vi "Write to Hardware.vi"(7 "Valid Triggers":bool, 8 "error in":errorcluster, 9 "Trigger Values":dbl[](array[numeric]), 10 "Values in":dbl[](array[numeric]), 11 "Tx Execution Unit Implementation in":refnum<class "Tx Generic Execution Unit.lvclass">) -> (0 "error out":errorcluster, 1 "Trigger Values out":dbl[](array[numeric]), 2 "Values out":dbl[](array[numeric]), 3 "Tx Execution Unit Implementation out":refnum<class "Tx Generic Execution Unit.lvclass">)   [LabVIEW 2020, in "AIM ARINC 664 Engine.lvlib" / "Implementation.lvlib" / "Tx Generic Execution Unit.lvclass"]
uses:
  Tx Generic Execution Unit.lvclass
  Tx Generic Execution Unit.lvclass/Tx Generic Execution Unit.ctl
  <instrlib>/AIM GmbH/_AIM 664/bsp/Fdx Stop (Tx).vi
  <instrlib>/AIM GmbH/_AIM 664/bsp/LIbraryAdmin/FdxGlobalDllPath.vi
  <instrlib>/AIM GmbH/_AIM 664/bsp/LIbraryAdmin/FdxGetErrorDescription.vi
  <vilib>/Utility/error.llb/Error Cluster From Error Code.vi
  <instrlib>/AIM GmbH/_AIM 664/AIM664LV.lvlib
  <vilib>/Utility/SystemLogging/NI_SystemLogging.lvlib
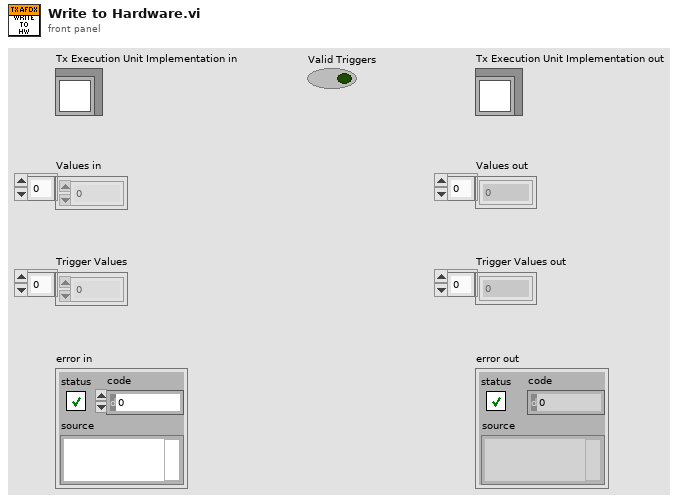
[diagram p1: front panel]
types:
  T1 = cluster{"StartMode":i32, "Count":u32, "Sign":i32, "Day":u32, "Hour":u32, "Min":u32, "Second":u32, "MilliSec":u32, "MicroSec":u32, "ExtendedStopMode":i32, "TransmitTime":u32}
  T2 = cluster{"Index":u32, "Offset":u32, "Lenght":u32, "SubQueueHandle":u32}
  T3 = typedef "Frame Payload Parameters.ctl" = cluster{"PayloadID":string, "FrameIndeces":u32[], "Parameters":cluster{"start index":i32, "size":i32, "encoding":T4, "signed":bool, "scale multiplier":dbl, "scale offset":dbl}[]}
  T4 = typedef "Encoding (Arinc664).ctl" = u16
  T5 = typedef "tx_generic_command.ctl" = enum16{"No Action", "Start", "Stop"}
  T6 = cluster{"start index":i32, "size":i32, "encoding":T4, "signed":bool, "scale multiplier":dbl, "scale offset":dbl}[]
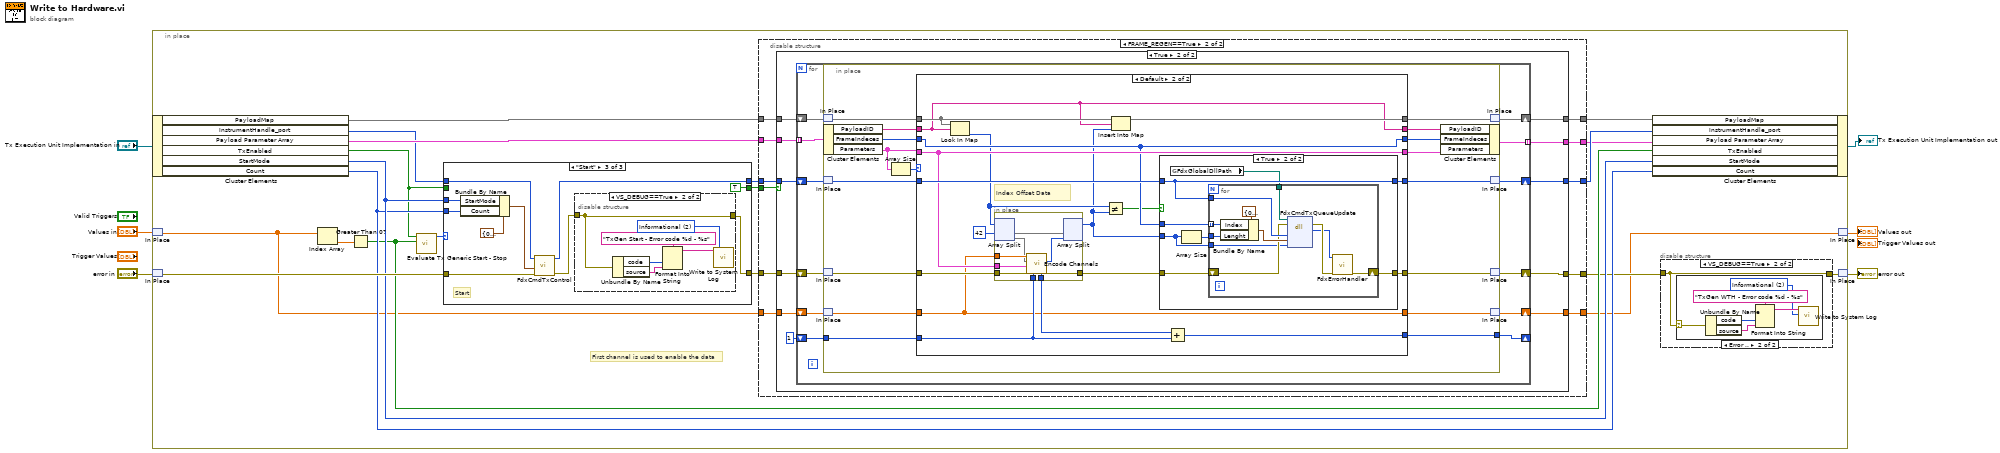
[diagram p0: block diagram]
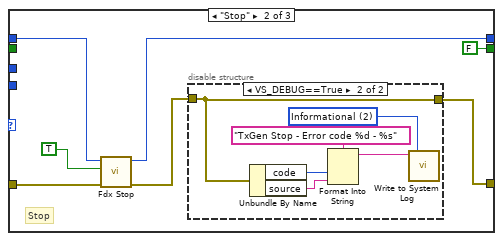
[diagram p5: hidden frame]
diagram:
  n1 = in-place {
    # "First channel is used to enable the data"
    n2 = in-place-cluster #1("Tx Execution Unit Implementation in") -> ("PayloadMap"=w8:map{string, u8[]}, "InstrumentHandle_port"=w22:u32, "Payload Parameter Array"=w26:T3[], "TxEnabled"=w11:bool, "StartMode"=w18:u32, "Count"=w17:u32)
    n3 = in-place-match #2("Values in") -> (w9:dbl[])
    n4 = in-place-match #3("error in") -> (w20:errorcluster)
    n5 = Index Array(array=w9) -> (element=w23:dbl)  [unwired: 1 in]
    n6 = Greater Than 0?(x=w23) -> (x > 0?=w15:bool)
    n7 = call "Evaluate Tx Generic Start - Stop.vi"("current"=w15, "last"=w11) -> ("tx generic command"=w16:T5)  [unwired: 9 in]
    n8 = case shown="\"Start\"" w16 {
      tunnel: w22 -> [w36 w41 w58]
      tunnel: w18 -> [_ _ w56]
      tunnel: w17 -> [_ _ w55]
      tunnel: w20 -> [w37 w43 w59]
      tunnel: [w37 w39 w53] -> w19
      tunnel: [w36 w42 w57] -> w21
      tunnel: w11 -> [w35 _ _]
      tunnel: [w35 FALSE ("TxEnabled") TRUE ("TxEnabled")] -> w10
      frame "No Action", Default {
      }
      frame "Stop" {
        # "Stop"
        n9 = call-poly <instrlib>:"Fdx Stop.vi"("error in"=w43, "Force Stop?"=TRUE, "InstrumentHandle_port in"=w41) -> ("error out"=w40:errorcluster, "InstrumentHandle_port out"=w42:u32)  [unwired: 7 in]
        n10 = disable-structure shown="VS_DEBUG==True" {
          disable-tunnel: w40 -> [w45 w46]
          disable-tunnel: [w45 w46] -> w39
          frame condition #0 {
          }
          frame condition #1 (active) {
            w49 = 2 items=["Error", "Warning", "Informational"] ("severity")
            n11 = Unbundle By Name(w46) -> ("code"=w48:i32, "source"=w47:string)
            n12 = Format Into String(format string="TxGen Stop - Error code %d - %s", w48, w47) -> (resulting string=w50:string)  [unwired: 2 in, 1 out]
            n13 = call <vilib>:"Write to System Log.vi"("severity"=w49, "message"=w50) -> ()  [unwired: 9 in, 1 out]
          }
        }
      }
      frame "Start" {
        # "Start"
        n14 = Bundle By Name(cluster=T1 {"StartMode"=0, "Count"=0, "Sign"=0, "Day"=0, "Hour"=0, "Min"=0, "Second"=0, "MilliSec"=0, "MicroSec"=0, "ExtendedStopMode"=0, "TransmitTime"=0} ("TxControl"), "StartMode"=w56, "Count"=w55) -> (w61:T1)
        n15 = call <instrlib>:"FdxCmdTxControl.vi"("error in"=w59, "TxControl"=w61, "InstrumentHandle_port in"=w58) -> ("error out"=w54:errorcluster, "InstrumentHandle_port out"=w57:u32)  [unwired: 7 in]
        n16 = disable-structure shown="VS_DEBUG==True" {
          disable-tunnel: w54 -> [w62 w63]
          disable-tunnel: [w62 w63] -> w53
          frame condition #0 {
          }
          frame condition #1 (active) {
            w66 = 2 items=["Error", "Warning", "Informational"] ("severity")
            n17 = Unbundle By Name(w63) -> ("code"=w65:i32, "source"=w64:string)
            n18 = Format Into String(format string="TxGen Start - Error code %d - %s", w65, w64) -> (resulting string=w67:string)  [unwired: 2 in, 1 out]
            n19 = call <vilib>:"Write to System Log.vi"("severity"=w66, "message"=w67) -> ()  [unwired: 9 in, 1 out]
          }
        }
      }
    }
    n20 = disable-structure shown="FRAME_REGEN==True" {
      disable-tunnel: w21 -> [w71 w81]
      disable-tunnel: w26 -> [w72 w79]
      disable-tunnel: w19 -> [w70 w83]
      disable-tunnel: [w70 w82] -> w14
      disable-tunnel: [w71 w80] -> w25
      disable-tunnel: [w72 w78] -> w24
      disable-tunnel: w9 -> [w69 w77]
      disable-tunnel: [w69 w76] -> w12
      disable-tunnel: w10 -> [_ w75]
      disable-tunnel: w8 -> [_ w74]
      disable-tunnel: [_ w73] -> w7
      frame condition #0 {
      }
      frame condition #1 (active) {
        n21 = case shown="True" w75 {
          tunnel: w83 -> [w86 w99]
          tunnel: [w86 w98] -> w82
          tunnel: w81 -> [w87 w97]
          tunnel: [w87 w96] -> w80
          tunnel: w79 -> [w88 w95]
          tunnel: [w88 w94] -> w78
          tunnel: w77 -> [w85 w89]
          tunnel: [w85 w93] -> w76
          tunnel: w74 -> [w84 w90]
          tunnel: [w84 w91] -> w73
          frame False {
          }
          frame True {
            n22 = for {
              shift-right: [w107] -> w98
              shift-left: w99 -> [w111]
              shift-right: [w104] -> w96
              shift-left: w97 -> [w110]
              tunnel: w95 -> [w109] mode=indexing
              tunnel: [w108] -> w94 mode=indexing
              shift-right: [w105] -> w93
              shift-left: w89 -> [w106]
              shift-right: [w103] -> _
              shift-left: 1 -> [w102]
              shift-right: [w101] -> w91
              shift-left: w90 -> [w100]
              n23 = in-place {
                in-place-border: [w125] -> w103
                in-place-border: w102 -> [w124]
                n24 = in-place-match #4(w100) -> (w121:map{string, u8[]})
                n25 = in-place-cluster #5(w109) -> ("PayloadID"=w119:string, "FrameIndeces"=w118:u32[], "Parameters"=w117:T6)
                n26 = in-place-match #6(w110) -> (w127:u32)
                n27 = in-place-match #7(w111) -> (w123:errorcluster)
                n28 = in-place-match #8(w106) -> (w126:dbl[])
                n29 = Array Size(array=w117) -> (size(s)=w122:i32)
                n30 = case shown="Default" w122 {
                  tunnel: [w136 w154] -> w128
                  tunnel: w127 -> [w134 w147]
                  tunnel: w126 -> [w129 w142]
                  tunnel: [w135 w152] -> w125
                  tunnel: w124 -> [w135 w151]
                  tunnel: w117 -> [w130 w144]
                  tunnel: w123 -> [w136 w150]
                  tunnel: w119 -> [w132 w143]
                  tunnel: w118 -> [w131 w140]
                  tunnel: w121 -> [w133 w146]
                  tunnel: [w134 w141] -> w120
                  tunnel: [w133 w145] -> w116
                  tunnel: [w131 w140] -> w115
                  tunnel: [w132 w143] -> w114
                  tunnel: [w130 w144] -> w113
                  tunnel: [w129 w142] -> w112
                  frame 0 {
                  }
                  frame Default {
                    # "Index Offset Data"
                    n31 = Look In Map(map=w146, key=w143) -> (value=w139:u8[])  [unwired: 1 in, 1 out]
                    n32 = in-place {
                      in-place-border: w142 -> [w183]
                      in-place-border: [w182] -> w153
                      in-place-border: w151 -> [w181]
                      in-place-border: w144 -> [w180]
                      in-place-border: w150 -> [w179]
                      in-place-border: [w178] -> w149
                      n33 = in-place-split #9(w139, 42) -> (w177:u8[], w176:u8[])
                      n34 = call "Encode Channels.vi"("Offset"=w181, "error in"=w179, "Parameters"=w180, "Data in"=w176, "Values in"=w183) -> ("error out"=w178:errorcluster, "Data out"=w175:u8[], "Number of Parameters"=w182:i32)  [unwired: 4 in]
                      n35 = in-place-split #9(w177, w175) -> (w138:u8[])  [unwired: 1 out]
                    }
                    n36 = Not Equal?(x=w139, y=w138) -> (x != y?=w137:bool)
                    n37 = Insert Into Map(map in=w146, key=w143, value=w138) -> (map out=w145:map{string, u8[]})  [unwired: 2 out]
                    n38 = case shown="True" w137 {
                      tunnel: [w155 w163] -> w154
                      tunnel: w149 -> [w155 w162]
                      tunnel: w147 -> [w156 w158]
                      tunnel: w140 -> [_ w160]
                      tunnel: w138 -> [_ w159]
                      tunnel: [w156 w158] -> w141
                      frame False {
                      }
                      frame True {
                        n39 = global read "FdxGlobalDllPath.vi" "FdxGlobalDllPath"() -> (w157:path)
                        n40 = Array Size(array=w159) -> (size(s)=w161:i32)
                        n41 = for {
                          tunnel: w158 -> [w169]
                          shift-right: [w174] -> w163
                          shift-left: w162 -> [w168]
                          tunnel: w160 -> [w167] mode=indexing
                          tunnel: w161 -> [w166]
                          tunnel: w159 -> [w165]
                          tunnel: w157 -> [w164]
                          n42 = Bundle By Name(cluster=T2 {"Index"=0, "Offset"=0, "Lenght"=0, "SubQueueHandle"=0}, "Index"=w167, "Lenght"=w166) -> (w172:T2)
                          n43 = dll-call lib="aim_fdx.19.dll" fn="FdxCmdTxQueueUpdate"(path in=w164, error in=w168, "InstrumentHandle"=w169, "TY_FDX_TX_QUEUE_UPDATEb"=w172, "WriteBuffer"=w165) -> (error out=w171:errorcluster, "status"=w170:i32)  [unwired: 3 in, 2 out]
                          n44 = call <instrlib>:"FdxErrorHandler.vi"("error in"=w171, "AIM Error"=w170) -> ("error out"=w174:errorcluster)  [unwired: 9 in]
                        }
                      }
                    }
                    n45 = Add(x=w153, y=w151) -> (x+y=w152:i32)
                  }
                }
                n46 = in-place-cluster #5("PayloadID"=w114, "FrameIndeces"=w115, "Parameters"=w113) -> (w108:T3)
                n47 = in-place-match #4(w116) -> (w101:map{string, u8[]})
                n48 = in-place-match #6(w120) -> (w104:u32)
                n49 = in-place-match #7(w128) -> (w107:errorcluster)
                n50 = in-place-match #8(w112) -> (w105:dbl[])
              }
            }
          }
        }
      }
    }
    n51 = in-place-cluster #1("PayloadMap"=w7, "InstrumentHandle_port"=w25, "Payload Parameter Array"=w24, "TxEnabled"=w15, "StartMode"=w18, "Count"=w17) -> (→"Tx Execution Unit Implementation out":refnum<class "Tx Generic Execution Unit.lvclass">)
    n52 = disable-structure shown="VS_DEBUG==True" {
      disable-tunnel: w14 -> [w27 w28]
      disable-tunnel: [w27 w28] -> w13
      frame condition #0 {
      }
      frame condition #1 (active) {
        n53 = case shown="Error .." w28 {
          selector: w28 -> [_ w29]
          frame No Error {
          }
          frame Error {
            w32 = 2 items=["Error", "Warning", "Informational"] ("severity")
            n54 = Unbundle By Name(w29) -> ("code"=w31:i32, "source"=w30:string)
            n55 = Format Into String(format string="TxGen WTH - Error code %d - %s", w31, w30) -> (resulting string=w33:string)  [unwired: 2 in, 1 out]
            n56 = call <vilib>:"Write to System Log.vi"("severity"=w32, "message"=w33) -> ()  [unwired: 9 in, 1 out]
          }
        }
      }
    }
    n57 = in-place-match #2(w12) -> (→"Values out":dbl[])
    n58 = in-place-match #3(w13) -> (→"error out":errorcluster)
  }
